vi "GetFastAlignmentInputID.vi"(0 "System no.":i32=1 min=1 max=4 step=1, 1 "Scan Name in":string, 2 "Fast Routine type":enum16{"FDG", "FDR"}(ring)=enum."FDR", 5 "error in":errorcluster) -> (14 "Analog channel out":i32, 19 "error out":errorcluster)   [LabVIEW 2020]
doc: "This VI reads all area scan rotuines from the controller and searches for the keyword \"A\" in the scan routine definition. The number after the keyword \"A\" is the fast alignment input ID."
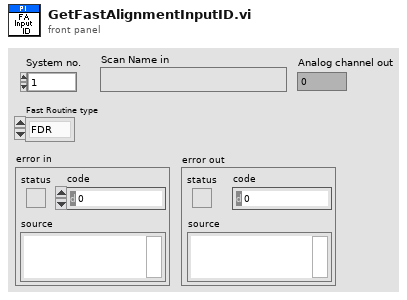
[diagram p1: front panel]
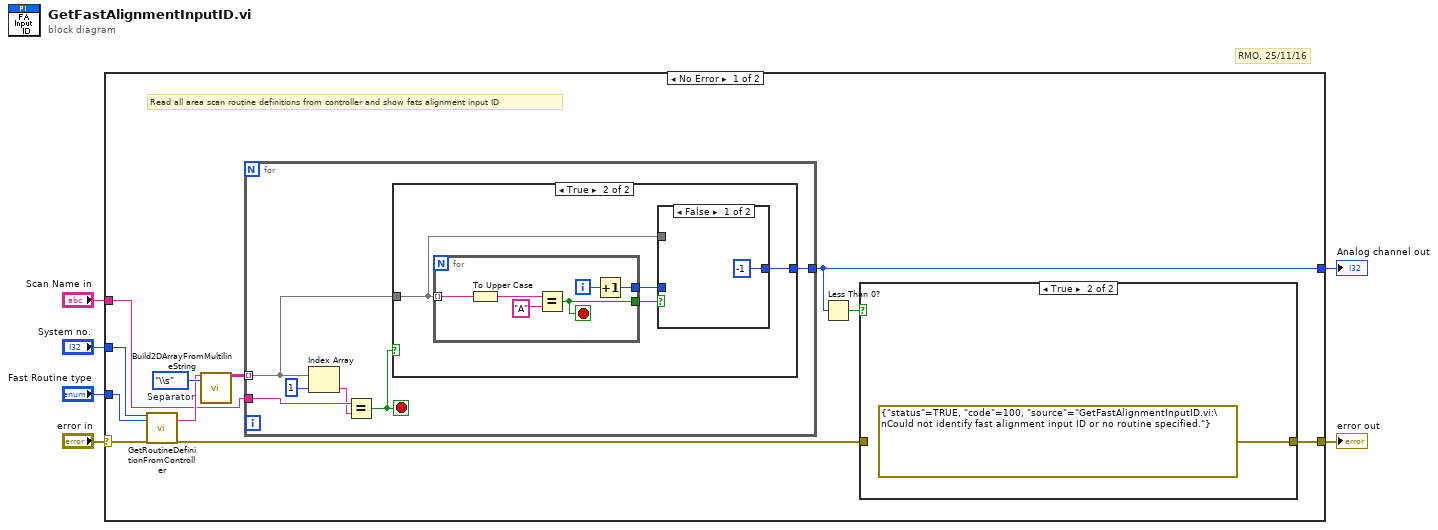
[diagram p0: block diagram]
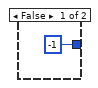
[diagram p3: hidden frame]
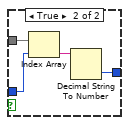
[diagram p4: hidden frame]
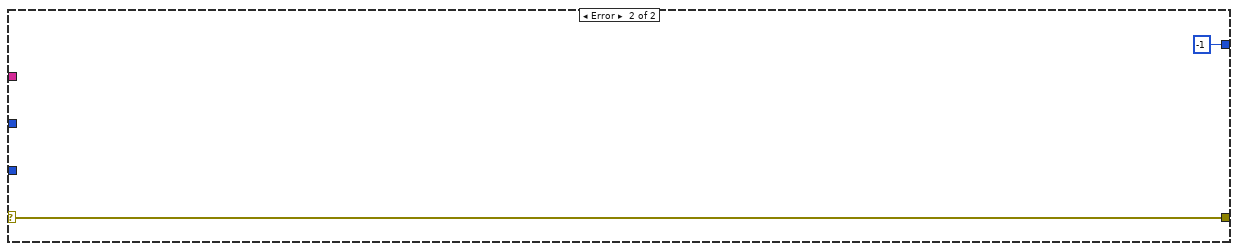
[diagram p5: hidden frame]
diagram:
  # "RMO, 25/11/16"
  n1 = case shown="No Error" "error in" {
    selector: "error in" -> [w16 w43]
    tunnel: [w8 w43] -> w6
    tunnel: "System no." -> [w14 _]
    tunnel: "Scan Name in" -> [w12 _]
    tunnel: [w11 -1] -> w2
    tunnel: "Fast Routine type" -> [w7 _]
    frame No Error {
      w17 = enum16{"\\s", "\\t"}."\\s"  # Separator
      # "Read all area scan routine definitions from controller and show fats alignment input ID"
      n2 = call "GetRoutineDefinitionFromController.vi"("System no."=w14, "Fast Routine type"=w7, "error in"=w16) -> ("Routine Definitons"=w13:string, "error out"=w9:errorcluster)  [unwired: 15 out]
      n3 = call "Build2DArrayFromMultilineString.vi"("String"=w13, "Separator"=w17) -> ("2D Array out"=w15:string[][])  [unwired: 17 out]
      n4 = for {
        tunnel: w15 -> [w21] mode=indexing
        tunnel: w12 -> [w24]
        tunnel: [w20] -> w11
        stop <- w22 stop-if-true
        n5 = Index Array(array=w21, index=1) -> (element=w23:string)
        n6 = Equal?(x=w24, y=w23) -> (x = y?=w22:bool)
        n7 = case shown="True" w22 {
          tunnel: w21 -> [_ w28]
          tunnel: [-1 w27] -> w20
          frame False {
          }
          frame True {
            n8 = for {
              tunnel: w28 -> [w39] mode=indexing
              tunnel: [w38] -> w30
              tunnel: [w36] -> w29
              i -> [w37]
              stop <- w38 stop-if-true
              n9 = To Upper Case(1:w39) -> (0:w41:string)
              n10 = Equal?(x=w41, y="A") -> (x = y?=w38:bool)
              n11 = Increment(x=w37) -> (x+1=w36:i32)
            }
            n12 = case shown="False" w30 {
              tunnel: w29 -> [_ w34]
              tunnel: w28 -> [_ w35]
              tunnel: [-1 w32] -> w27
              frame False {
              }
              frame True {
                n13 = Index Array(array=w35, index=w34) -> (element=w33:string)
                n14 = Decimal String To Number(string=w33) -> (number=w32:i32)  [unwired: 3 out]
              }
            }
          }
        }
      }
      n15 = Less Than 0?(x=w11) -> (x < 0?=w10:bool)
      n16 = case shown="True" w10 {
        tunnel: w9 -> [w18 _]
        tunnel: [w18 errorcluster {"status"=TRUE, "code"=100, "source"="GetFastAlignmentInputID.vi:\nCould not identify fast alignment input ID or no routine specified."} ("error out")] -> w8
        frame False {
        }
        frame True {
        }
      }
    }
    frame Error {
    }
  }
  "error out" <- w6
  "Analog channel out" <- w2
